vi "Caller Queue .vi"(8 "error in (no error)":errorcluster, 10 "Cluster":T1, 11 "Module Number  3":dbl=1.0) -> (0 "error out":errorcluster)   [LabVIEW 2015, in "Copy of Untitled Library 1.lvlib"]
uses:
  Copy of Untitled Library 1.lvlib
  Controls/Caller Queue Control .ctl
  Controls/Control 1.ctl
  Controls/Enum Constant.ctl
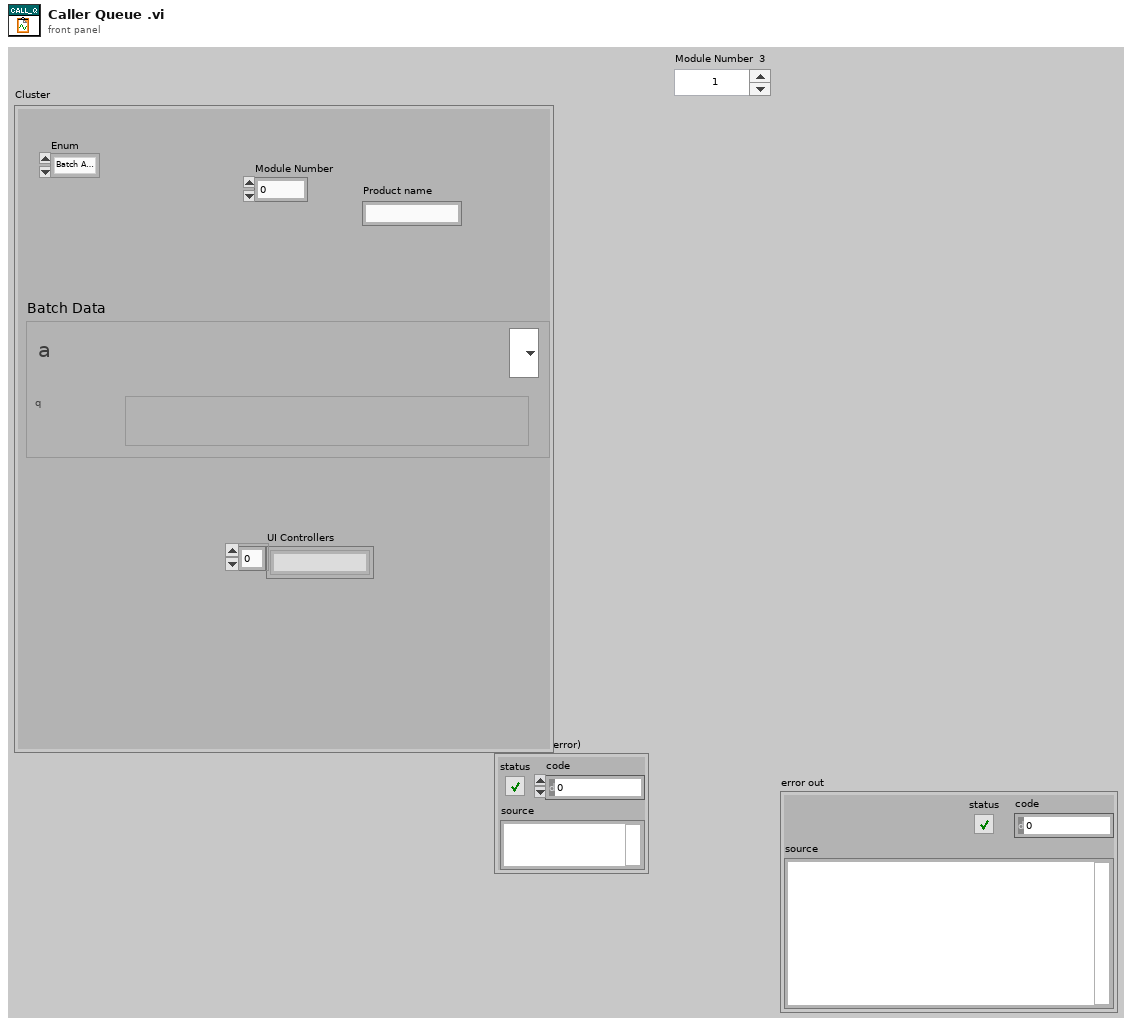
[diagram p1: front panel]
types:
  T1 = typedef "Caller Queue Control .ctl" = cluster{"Enum":enum16{"Batch Added", "Batch Deleted", "Batch Opened", "Batch Closed", "Batch Edited", "new Product Added", "Product deleted "}, "Batch Data 3":T2, "UI Controllers":string[], "Product name":string, "Module Number":dbl}
  T2 = typedef "Copy of Untitled Library 1.lvlib/Control 1.ctl" = cluster{"DATA":string, "DATA 2":string, "DATA 3":string, "DATA 4":string, "DATA 5":string, "DATA 6":string, "DATA 7":string, "DATA 8":string, "DATA 9":string, "DATA 10":string, "Product":string}
  T3 = typedef "Enum Constant.ctl" = enum16{"Init", "Read", "Write"}
  T4 = typedef "FGV Data.ctl" = T5[]
  T5 = typedef "FGV Cluster Data.ctl" = cluster{"Manual/Automatic":bool, "UI Controllers ":string[], "UI Primery Key ":dbl[], "Caller Queue & MSG":T6, "Module ID":dbl, "DB Reference In":T7, "Products Columns":string[], "Cluster":cluster{"Delete Product":enum8{"Enabled", "Disabled", "Disabled and Grayed Out"}, "Add Product ":enum8{"Enabled", "Disabled", "Disabled and Grayed Out"}, "EDIT BATCH":enum8{"Enabled", "Disabled", "Disabled and Grayed Out"}, "Open Batch ":enum8{"Enabled", "Disabled", "Disabled and Grayed Out"}, "Close Batch":enum8{"Enabled", "Disabled", "Disabled and Grayed Out"}, "Delete Batch":enum8{"Enabled", "Disabled", "Disabled and Grayed Out"}, "Add Batch ":enum8{"Enabled", "Disabled", "Disabled and Grayed Out"}}}
  T6 = typedef "Queue and Caller MSG.ctl" = cluster{"Caller Queue":refnum<queue>, "Caller MSG":string}
  T7 = typedef "NI_Database_API.lvlib/Conn ObjectReference.ctl" = refnum<k1>
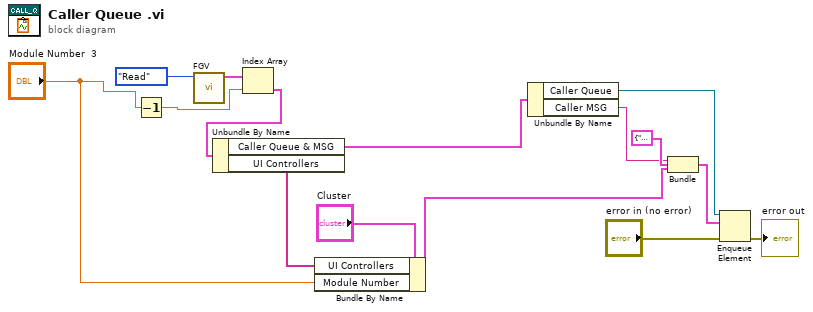
[diagram p0: block diagram]
diagram:
  n1 = Decrement(x="Module Number  3") -> (x-1=w6:dbl)
  n2 = call "FGV.vi"("Enum"=Enum_Constant."Read") -> ("Read Data"=w8:T4)  [unwired: 9 in, 1 out]
  n3 = Index Array(array=w8, index=w6) -> (element=w9:T5)
  n4 = Unbundle By Name(w9) -> ("Caller Queue & MSG"=w5:T6, "UI Controllers"=w3:string[])
  n5 = Bundle By Name(cluster="Cluster", "UI Controllers"=w3, "Module Number"="Module Number  3") -> (w2:T1)
  n6 = Unbundle By Name(w5) -> ("Caller Queue"=w15:refnum<queue>, "Caller MSG"=w13:string)
  n7 = Bundle(cluster=cluster{string, variant} {"", variant}, w13, w2) -> (w12:cluster{string, variant})
  n8 = Enqueue Element(queue=w15, element=w12, error in (no error)="error in (no error)") -> (error out=→"error out":errorcluster)  [unwired: 1 in, 2 out]
